vi "Getprofile.vi"(8 "error in (no error)":errorcluster, 10 "Array":dbl[](array[numeric]), 11 "Refnum in":T1) -> (0 "error out":errorcluster, 3 "Pixels Line":sgl[](array[numeric]))   [LabVIEW 2015]
uses:
  <vilib>/vision/Image Controls.llb/IMAQ Image.ctl
  <vilib>/vision/NI_Vision_Development_Module.lvlib
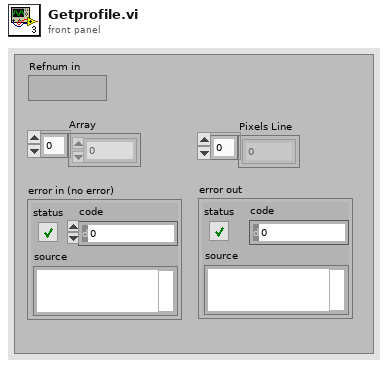
[diagram p1: front panel]
types:
  T1 = typedef "IMAQ Image.ctl" = refnum<image>
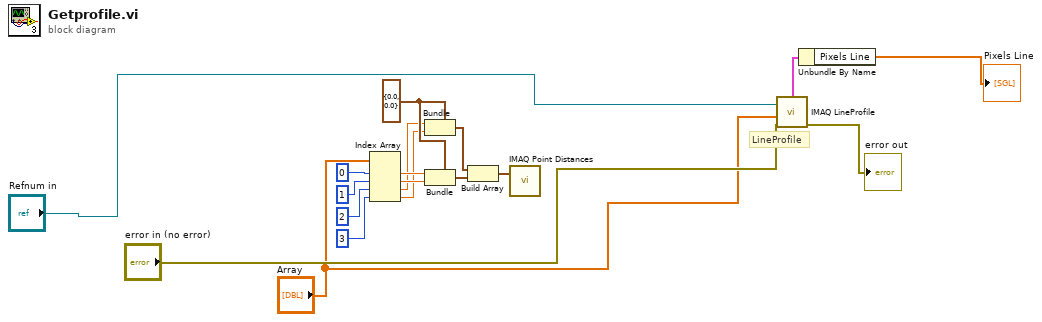
[diagram p0: block diagram]
diagram:
  w6 = cluster{"X":sgl, "Y":sgl} {"X"=0.0, "Y"=0.0}
  # "LineProfile"
  n1 = Index Array(array="Array", index #1=0 ("index"), index #2=1 ("index"), index #3=2 ("index"), index #4=3 ("index")) -> (element #1=w5:dbl, element #2=w4:dbl, element #3=w3:dbl, element #4=w2:dbl)
  n2 = Bundle(cluster=w6, "X"=w3, "Y"=w2) -> (w7:cluster{"X":sgl, "Y":sgl})
  n3 = Bundle(cluster=w6, "X"=w5, "Y"=w4) -> (w8:cluster{"X":sgl, "Y":sgl})
  n4 = Build Array(w7, w8) -> (w9:cluster{"X":sgl, "Y":sgl}[])
  n5 = call "IMAQ Point Distances"("Points"=w9) -> ()  [unwired: 4 in, 2 out]
  n6 = call "IMAQ LineProfile"("error in (no error)"="error in (no error)", "Line Coordinates"="Array", "Image"="Refnum in") -> ("error out"=→"error out":errorcluster, "Line Graph"=w14:cluster{"x0":sgl, "dx":sgl, "Pixels Line":sgl[]})  [unwired: 4 out]
  n7 = Unbundle By Name(w14) -> ("Pixels Line"=→"Pixels Line":sgl[])
